vi "Cube Manipulation Logic Core.vi"(6 "Auto Control":bool, 8 "Manual Intake Control":dbl, 10 "Manual Lift Control":dbl, 11 "Cube Manipulation Button Controls":T3) -> (0 "Safety Limit Engaged":bool, 3 "output cluster":T1={"Control Mode"=1, "Carrage Output"=0.0, "Intake Output"=0.0, "Intake Short"=FALSE, "Intake Long"=FALSE, "Lift Output"=0.0} {"Control Mode" items=["PercentOutput"=0, "Position"=1, "Velocity"=2, "Current"=3, "Follower"=5, "MotionProfile"=6, "MotionMagic"=7, "MotionMagicArc"=8, "MotionProfileArc"=10, "Disabled"=15]}, 5 "Sequence Done":bool, 7 "Position Reached":bool)   [LabVIEW 2017]
uses:
  Cube Manipulation Controls.ctl
  Cube Manipulation Outputs.ctl
  <vilib>/Rock Robotics/WPI/ThirdParty/Phoenix-LabVIEW/Motor Controller/Controls/CTRE_Phoenix_MotorControl_ControlMode.ctl
  Robot Global Data.vi
panel:
  in  "Intake Output":dbl=0.75 format="%#_13g"
  in  "y":dbl=-3500.0 format="%#_13g"
  in  "Exchange Sequence":dbl
  in  "Trigger Offset":dbl=5000.0
  in  "Command":dbl
  in  "Sequence Position":dbl
  # "Off= Retracted\nOn= Extended"
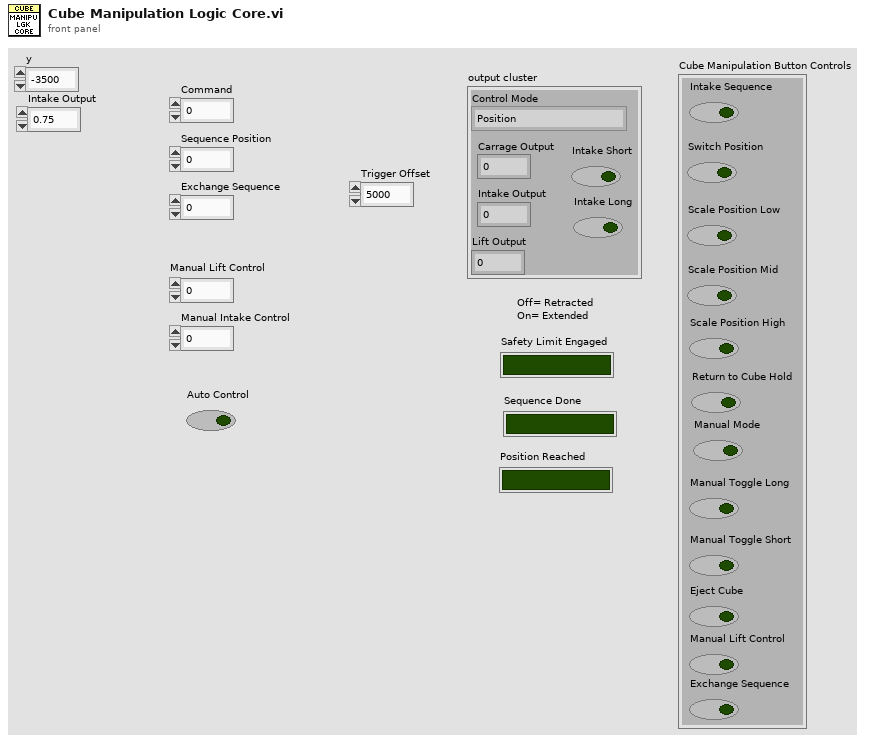
[diagram p1: front panel]
types:
  T1 = typedef "Cube Manipulation Outputs.ctl" = cluster{"Control Mode":T2, "Carrage Output":dbl, "Intake Output":dbl, "Intake Short":bool, "Intake Long":bool, "Lift Output":dbl}
  T2 = typedef "CTRE_Phoenix_MotorControl_ControlMode.ctl" = u16
  T3 = typedef "Cube Manipulation Controls.ctl" = cluster{"Intake Sequence":bool, "Switch Position":bool, "Scale Position Low":bool, "Scale Position Mid":bool, "Scale Position High":bool, "Return to Cube Hold":bool, "Manual Mode":bool, "Manual Toggle Long":bool, "Manual Toggle Short":bool, "Eject Cube":bool, "Manual Lift Control":bool, "Exchange Sequence":bool}
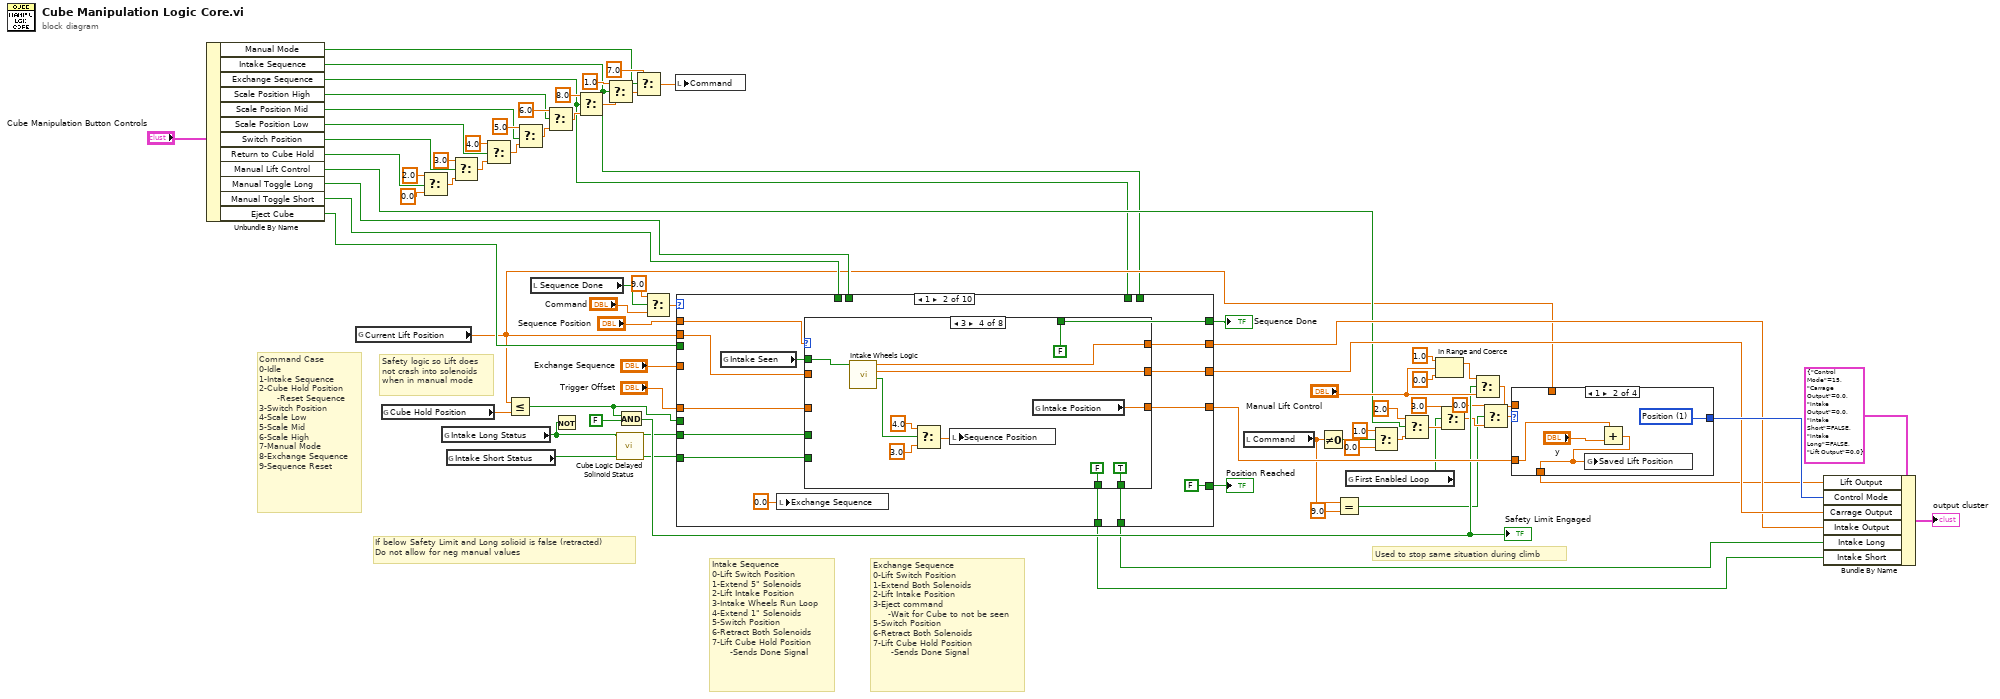
[diagram p0: block diagram]
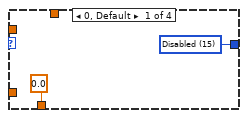
[diagram p2: hidden frame]
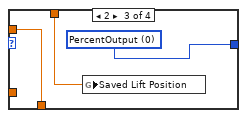
[diagram p3: hidden frame]
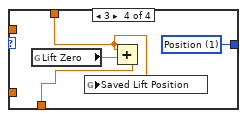
[diagram p4: hidden frame]
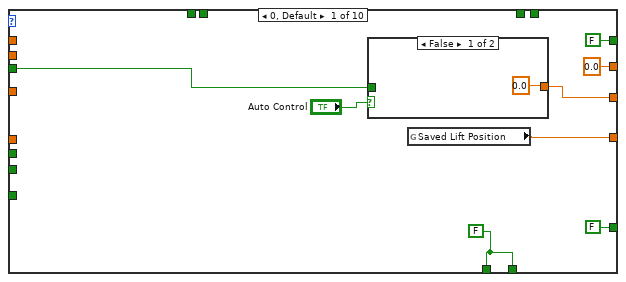
[diagram p5: hidden frame]
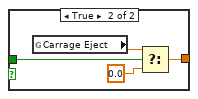
[diagram p6: hidden frame]
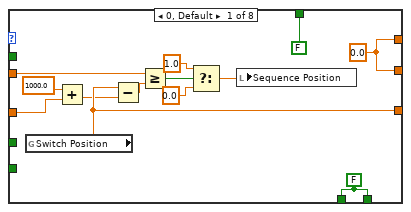
[diagram p7: hidden frame]
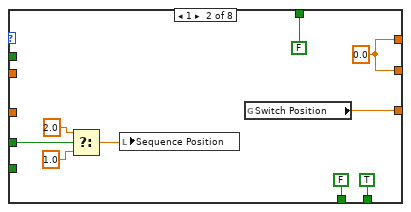
[diagram p8: hidden frame]
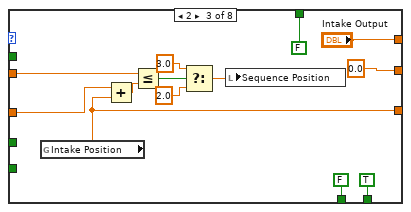
[diagram p9: hidden frame]
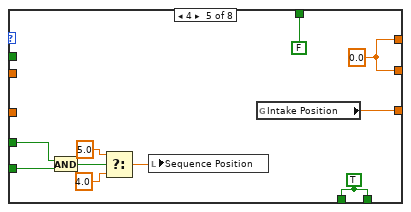
[diagram p10: hidden frame]
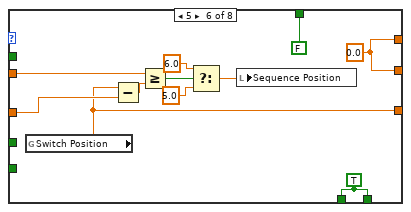
[diagram p11: hidden frame]
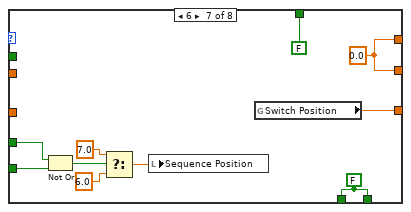
[diagram p12: hidden frame]
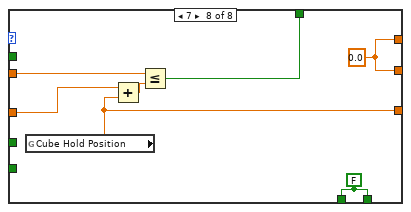
[diagram p13: hidden frame]
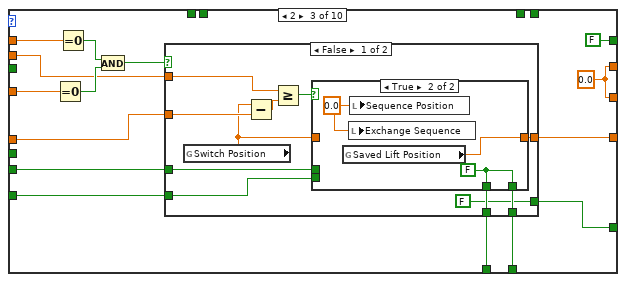
[diagram p14: hidden frame]
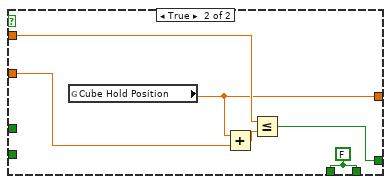
[diagram p16: hidden frame]
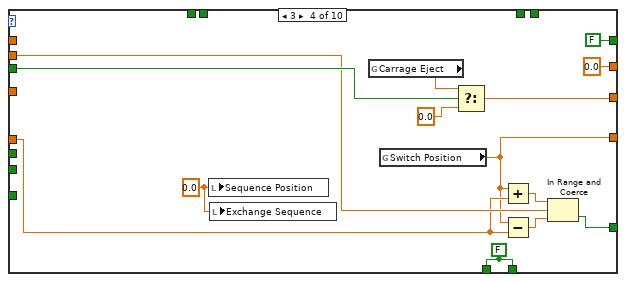
[diagram p17: hidden frame]
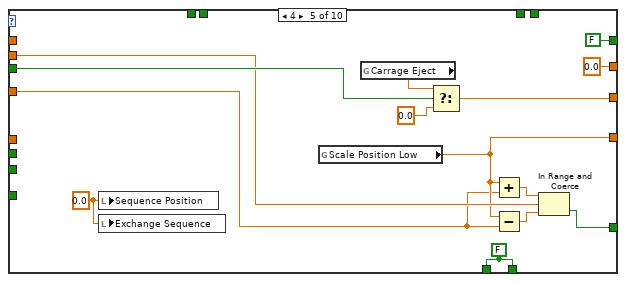
[diagram p18: hidden frame]
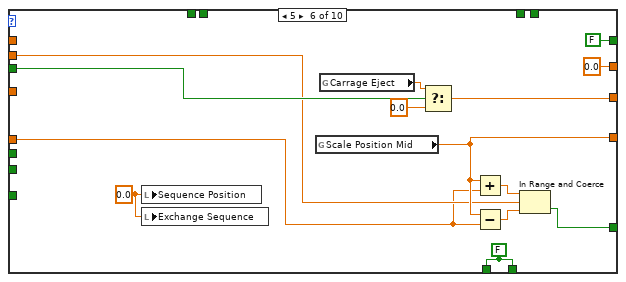
[diagram p19: hidden frame]
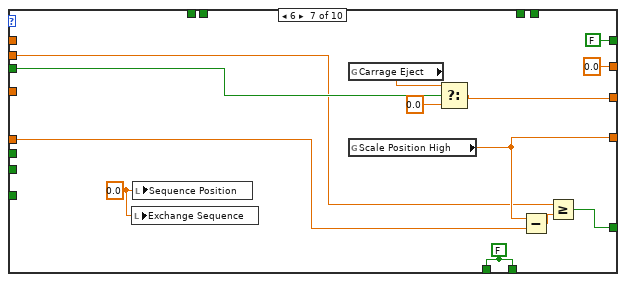
[diagram p20: hidden frame]
diagram:
  # "Used to stop same situation during climb"
  # "Exchange Sequence\n0-Lift Switch Position\n1-Extend Both Solenoids\n2-Lift Intake Position\n3-Eject command\n     -Wait for Cube to not be seen\n5-Switch Position\n6-Retract Both Solenoids\n7-Lift Cube Hold Position\n      -Sends Done Signal"
  # "If below Safety Limit and Long solioid is false (retracted)\nDo not allow for neg manual values"
  # "Command Case\n0-Idle\n1-Intake Sequence\n2-Cube Hold Position\n      -Reset Sequence\n3-Switch Position\n4-Scale Low\n5-Scale Mid\n6-Scale High\n7-Manual Mode\n8-Exchange Sequence\n9-Sequence Reset"
  # "Safety logic so Lift does\nnot crash into solenoids\nwhen in manual mode"
  # "Intake Sequence\n0-Lift Switch Position\n1-Extend 5\" Solenoids\n2-Lift Intake Position\n3-Intake Wheels Run Loop\n4-Extend 1\" Solenoids\n5-Switch Position\n6-Retract Both Solenoids\n7-Lift Cube Hold Position\n      -Sends Done Signal"
  n1 = Unbundle By Name("Cube Manipulation Button Controls") -> ("Manual Mode"=w29:bool, "Intake Sequence"=w21:bool, "Exchange Sequence"=w20:bool, "Scale Position High"=w45:bool, "Scale Position Mid"=w46:bool, "Scale Position Low"=w47:bool, "Switch Position"=w48:bool, "Return to Cube Hold"=w49:bool, "Manual Lift Control"=w34:bool, "Manual Toggle Long"=w36:bool, "Manual Toggle Short"=w35:bool, "Eject Cube"=w37:bool)
  n2 = global read "Robot Global Data.vi" "Current Lift Position"() -> (w33:dbl)
  n3 = global read "Robot Global Data.vi" "Cube Hold Position"() -> (w8:dbl)
  n4 = Select(t=2.0, s=w49, f=0.0) -> (s? t:f=w73:dbl)
  n5 = global read "Robot Global Data.vi" "Intake Long Status"() -> (w15:bool)
  n6 = global read "Robot Global Data.vi" "Intake Short Status"() -> (w14:bool)
  n7 = Select(t=3.0, s=w48, f=w73) -> (s? t:f=w74:dbl)
  n8 = Select(t=4.0, s=w47, f=w74) -> (s? t:f=w75:dbl)
  n9 = Less Or Equal?(x=w33, y=w8) -> (x <= y?=w9:bool)
  n10 = Select(t=5.0, s=w46, f=w75) -> (s? t:f=w72:dbl)
  n11 = local read "Sequence Done"() -> (w23:bool)
  n12 = Select(t=6.0, s=w45, f=w72) -> (s? t:f=w76:dbl)
  n13 = Not(x=w15) -> ()  [unwired: 1 out]
  n14 = Select(t=8.0, s=w20, f=w76) -> (s? t:f=w59:dbl)
  n15 = Select(t=1.0, s=w21, f=w59) -> (s? t:f=w32:dbl)
  n16 = call "Cube Logic Delayed Solinoid Status.vi"("Short Input"=w14, "Long Input"=w15) -> ("Short Delayed Output"=w16:bool, "Long Delayed Output"=w17:bool)  [unwired: 8 in]
  n17 = And(x=w9, y=FALSE) -> (x .and. y?=w44:bool)
  "Safety Limit Engaged" <- w44
  n18 = Select(t=7.0, s=w29, f=w32) -> (s? t:f=w31:dbl)
  n19 = Select(t=9.0, s=w23, f="Command") -> (s? t:f=w25:dbl)
  n20 = local write "Command"(w31) -> ()
  n21 = case shown="1" w25 {
    tunnel: w33 -> [_ w103 w190 w232 w244 w257 w270 _ w322 _]
    tunnel: [w81 w102 w196 w228 w243 w258 w272 w286 w321 w400] -> w57
    tunnel: [w77 w101 w195 w239 w253 w267 w280 w300 w320 w407] -> w19
    tunnel: [w77 w100 w194 w239 w253 w267 w280 w301 w319 w406] -> w18
    tunnel: w17 -> [_ w99 w192 _ _ _ _ _ w318 w407]
    tunnel: [0.0 ("Intake Output") w98 w188 0.0 ("Intake Output") 0.0 ("Intake Output") 0.0 ("Intake Output") 0.0 ("Intake Output") w297 w317 w399] -> w40
    tunnel: [w80 w97 w188 w237 w252 w266 w278 w299 w316 w399] -> w41
    tunnel: w16 -> [_ w95 w193 _ _ _ _ _ w315 w406]
    tunnel: "Sequence Position" -> [_ w94 w200 _ _ _ _ _ _ _]
    tunnel: w37 -> [w79 _ _ w238 w251 w264 w277 _ w309 _]
    tunnel: w36 -> [_ _ _ _ _ _ _ w282 _ _]
    tunnel: w35 -> [_ _ _ _ _ _ _ w281 _ _]
    tunnel: "Trigger Offset" -> [_ w93 w191 w229 _ w256 w271 _ w314 _]
    tunnel: "Exchange Sequence" -> [_ _ w201 _ w242 _ _ _ w313 _]
    tunnel: [FALSE w92 FALSE FALSE FALSE FALSE FALSE FALSE w312 w404] -> w26
    tunnel: w21 -> [_ _ _ _ _ _ _ _ _ w403]
    tunnel: w20 -> [_ _ _ _ _ _ _ _ _ w402]
    tunnel: [FALSE FALSE w189 w233 w245 w259 w273 FALSE FALSE FALSE] -> w13
    tunnel: w9 -> [_ _ _ _ _ _ _ _ _ _]
    frame 0, Default {
      w77 = FALSE
      n22 = case shown="False" "Auto Control" {
        tunnel: [0.0 w87] -> w80
        tunnel: w79 -> [_ w86]
        frame False {
        }
        frame True {
          n23 = global read "Robot Global Data.vi" "Carrage Eject"() -> (w89:dbl)
          n24 = Select(t=w89, s=w86, f=0.0) -> (s? t:f=w87:dbl)
        }
      }
      n25 = global read "Robot Global Data.vi" "Saved Lift Position"() -> (w81:dbl)
    }
    frame 1 {
      n26 = global read "Robot Global Data.vi" "Intake Seen"() -> (w96:bool)
      n27 = local write "Exchange Sequence"(0.0 ("Exchange Sequence")) -> ()
      n28 = case shown="3" w94 {
        tunnel: w103 -> [w116 _ w133 _ _ w170 _ w187]
        tunnel: [w109 w125 w130 w147 w159 w163 w180 w184] -> w102
        tunnel: w93 -> [w110 _ w129 _ _ w164 _ w183]
        tunnel: [w108 TRUE TRUE TRUE w158 w162 w179 w185] -> w101
        tunnel: [w108 FALSE FALSE FALSE w158 w162 w179 w185] -> w100
        tunnel: w99 -> [_ w120 _ _ w153 _ w173 _]
        tunnel: [w106 w117 "Intake Output" w142 w150 w160 w171 w181] -> w98
        tunnel: [w106 w117 0.0 ("Intake Output") w141 w150 w160 w171 w181] -> w97
        tunnel: w96 -> [_ _ _ w140 _ _ _ _]
        tunnel: w95 -> [_ _ _ _ w152 _ w175 _]
        tunnel: [FALSE FALSE FALSE FALSE FALSE FALSE FALSE w182] -> w92
        frame 0, Default {
          w106 = 0.0 ("Intake Output")
          w108 = FALSE
          n29 = global read "Robot Global Data.vi" "Switch Position"() -> (w109:dbl)
          n30 = Add(x=1000.0, y=w110) -> (x+y=w105:dbl)
          n31 = Subtract(x=w109, y=w105) -> (x-y=w111:dbl)
          n32 = Greater Or Equal?(x=w116, y=w111) -> (x >= y?=w115:bool)
          n33 = Select(t=1.0, s=w115, f=0.0) -> (s? t:f=w112:dbl)
          n34 = local write "Sequence Position"(w112) -> ()
        }
        frame 1 {
          w117 = 0.0 ("Intake Output")
          n35 = Select(t=2.0, s=w120, f=1.0) -> (s? t:f=w119:dbl)
          n36 = local write "Sequence Position"(w119) -> ()
          n37 = global read "Robot Global Data.vi" "Switch Position"() -> (w125:dbl)
        }
        frame 2 {
          n38 = global read "Robot Global Data.vi" "Intake Position"() -> (w130:dbl)
          n39 = Add(x=w129, y=w130) -> (x+y=w134:dbl)
          n40 = Less Or Equal?(x=w133, y=w134) -> (x <= y?=w136:bool)
          n41 = Select(t=3.0, s=w136, f=2.0) -> (s? t:f=w131:dbl)
          n42 = local write "Sequence Position"(w131) -> ()
        }
        frame 3 {
          n43 = call "Intake Wheels Logic.vi"("Intake Seen"=w140) -> ("Done"=w144:bool, "Carrage Output"=w141:dbl, "Intake Output"=w142:dbl)  [unwired: 8 in]
          n44 = Select(t=4.0, s=w144, f=3.0) -> (s? t:f=w143:dbl)
          n45 = local write "Sequence Position"(w143) -> ()
          n46 = global read "Robot Global Data.vi" "Intake Position"() -> (w147:dbl)
        }
        frame 4 {
          w158 = TRUE
          w150 = 0.0 ("Intake Output")
          n47 = And(x=w153, y=w152) -> (x .and. y?=w154:bool)
          n48 = Select(t=5.0, s=w154, f=4.0) -> (s? t:f=w155:dbl)
          n49 = local write "Sequence Position"(w155) -> ()
          n50 = global read "Robot Global Data.vi" "Intake Position"() -> (w159:dbl)
        }
        frame 5 {
          w160 = 0.0 ("Intake Output")
          w162 = TRUE
          n51 = global read "Robot Global Data.vi" "Switch Position"() -> (w163:dbl)
          n52 = Subtract(x=w163, y=w164) -> (x-y=w165:dbl)
          n53 = Greater Or Equal?(x=w170, y=w165) -> (x >= y?=w169:bool)
          n54 = Select(t=6.0, s=w169, f=5.0) -> (s? t:f=w166:dbl)
          n55 = local write "Sequence Position"(w166) -> ()
        }
        frame 6 {
          w179 = FALSE
          w171 = 0.0 ("Intake Output")
          n56 = Not Or(1:w175, 2:w173) -> (0:w174:bool)
          n57 = Select(t=7.0, s=w174, f=6.0) -> (s? t:f=w176:dbl)
          n58 = local write "Sequence Position"(w176) -> ()
          n59 = global read "Robot Global Data.vi" "Switch Position"() -> (w180:dbl)
        }
        frame 7 {
          w181 = 0.0 ("Intake Output")
          w185 = FALSE
          n60 = global read "Robot Global Data.vi" "Cube Hold Position"() -> (w184:dbl)
          n61 = Add(x=w183, y=w184) -> (x+y=w186:dbl)
          n62 = Less Or Equal?(x=w187, y=w186) -> (x <= y?=w182:bool)
        }
      }
    }
    frame 2 {
      w188 = 0.0 ("Intake Output")
      n63 = Equal To 0?(x=w201) -> (x = 0?=w198:bool)
      n64 = Equal To 0?(x=w200) -> (x = 0?=w199:bool)
      n65 = And(x=w199, y=w198) -> (x .and. y?=w197:bool)
      n66 = case shown="False" w197 {
        tunnel: [w206 w222] -> w196
        tunnel: [w208 w225] -> w195
        tunnel: [w209 w225] -> w194
        tunnel: w193 -> [w205 _]
        tunnel: w192 -> [w204 _]
        tunnel: w191 -> [w212 w221]
        tunnel: w190 -> [w211 w223]
        tunnel: [FALSE w220] -> w189
        frame False {
          n67 = global read "Robot Global Data.vi" "Switch Position"() -> (w207:dbl)
          n68 = Subtract(x=w207, y=w212) -> (x-y=w213:dbl)
          n69 = Greater Or Equal?(x=w211, y=w213) -> (x >= y?=w210:bool)
          n70 = case shown="True" w210 {
            tunnel: [w215 w219] -> w209
            tunnel: [w214 w219] -> w208
            tunnel: w207 -> [w216 _]
            tunnel: [w216 w217] -> w206
            tunnel: w205 -> [w215 _]
            tunnel: w204 -> [w214 _]
            frame False {
            }
            frame True {
              w218 = 0.0 ("Sequence Position")
              w219 = FALSE
              n71 = global read "Robot Global Data.vi" "Saved Lift Position"() -> (w217:dbl)
              n72 = local write "Exchange Sequence"(w218) -> ()
              n73 = local write "Sequence Position"(w218) -> ()
            }
          }
        }
        frame True {
          w225 = FALSE
          n74 = global read "Robot Global Data.vi" "Cube Hold Position"() -> (w222:dbl)
          n75 = Add(x=w222, y=w221) -> (x+y=w224:dbl)
          n76 = Less Or Equal?(x=w223, y=w224) -> (x <= y?=w220:bool)
        }
      }
    }
    frame 3 {
      w234 = 0.0 ("Sequence Position")
      w239 = FALSE
      n77 = local write "Sequence Position"(w234) -> ()
      n78 = local write "Exchange Sequence"(w234) -> ()
      n79 = global read "Robot Global Data.vi" "Carrage Eject"() -> (w226:dbl)
      n80 = global read "Robot Global Data.vi" "Switch Position"() -> (w228:dbl)
      n81 = Select(t=w226, s=w238, f=0.0 ("t")) -> (s? t:f=w237:dbl)
      n82 = Add(x=w228, y=w229) -> (x+y=w231:dbl)
      n83 = Subtract(x=w228, y=w229) -> (x-y=w230:dbl)
      n84 = In Range and Coerce(upper limit=w231, x=w232, lower limit=w230) -> (In Range?=w233:bool)  [unwired: 1 out]
    }
    frame 4 {
      w248 = 0.0 ("Sequence Position")
      w253 = FALSE
      n85 = local write "Sequence Position"(w248) -> ()
      n86 = local write "Exchange Sequence"(w248) -> ()
      n87 = global read "Robot Global Data.vi" "Scale Position Low"() -> (w243:dbl)
      n88 = global read "Robot Global Data.vi" "Carrage Eject"() -> (w240:dbl)
      n89 = Select(t=w240, s=w251, f=0.0 ("t")) -> (s? t:f=w252:dbl)
      n90 = Add(x=w243, y=w242) -> (x+y=w247:dbl)
      n91 = Subtract(x=w243, y=w242) -> (x-y=w246:dbl)
      n92 = In Range and Coerce(upper limit=w247, x=w244, lower limit=w246) -> (In Range?=w245:bool)  [unwired: 1 out]
    }
    frame 5 {
      w262 = 0.0 ("Sequence Position")
      w267 = FALSE
      n93 = local write "Sequence Position"(w262) -> ()
      n94 = local write "Exchange Sequence"(w262) -> ()
      n95 = global read "Robot Global Data.vi" "Scale Position Mid"() -> (w258:dbl)
      n96 = global read "Robot Global Data.vi" "Carrage Eject"() -> (w255:dbl)
      n97 = Select(t=w255, s=w264, f=0.0) -> (s? t:f=w266:dbl)
      n98 = Add(x=w258, y=w256) -> (x+y=w261:dbl)
      n99 = Subtract(x=w258, y=w256) -> (x-y=w260:dbl)
      n100 = In Range and Coerce(upper limit=w261, x=w257, lower limit=w260) -> (In Range?=w259:bool)  [unwired: 1 out]
    }
    frame 6 {
      w275 = 0.0 ("Sequence Position")
      w280 = FALSE
      n101 = local write "Exchange Sequence"(w275) -> ()
      n102 = local write "Sequence Position"(w275) -> ()
      n103 = global read "Robot Global Data.vi" "Carrage Eject"() -> (w269:dbl)
      n104 = global read "Robot Global Data.vi" "Scale Position High"() -> (w272:dbl)
      n105 = Select(t=w269, s=w277, f=0.0) -> (s? t:f=w278:dbl)
      n106 = Subtract(x=w272, y=w271) -> (x-y=w274:dbl)
      n107 = Greater Or Equal?(x=w270, y=w274) -> (x >= y?=w273:bool)
    }
    frame 7 {
      w288 = 0.0 ("Sequence Position")
      # "Long"
      # "Short"
      n108 = local write "Sequence Position"(w288) -> ()
      n109 = local write "Exchange Sequence"(w288) -> ()
      n110 = case shown="False" w281 {
        tunnel: [w305 w306] -> w301
        frame False {
          n111 = global read "Robot Global Data.vi" "Intake Short Status"() -> (w305:bool)
        }
        frame True {
          n112 = global read "Robot Global Data.vi" "Intake Short Status"() -> (w307:bool)
          n113 = Not(x=w307) -> (.not. x?=w306:bool)
          n114 = global write "Robot Global Data.vi" "Intake Short Status"(w306) -> ()
        }
      }
      n115 = case shown="True" w282 {
        tunnel: [w302 w303] -> w300
        frame False {
          n116 = global read "Robot Global Data.vi" "Intake Long Status"() -> (w302:bool)
        }
        frame True {
          n117 = global read "Robot Global Data.vi" "Intake Long Status"() -> (w304:bool)
          n118 = Not(x=w304) -> (.not. x?=w303:bool)
          n119 = global write "Robot Global Data.vi" "Intake Long Status"(w303) -> ()
        }
      }
      n120 = Less?(x="Manual Intake Control", y=-0.25) -> (x < y?=w293:bool)
      n121 = Greater?(x="Manual Intake Control", y=0.25) -> (0:w294:bool)
      n122 = global read "Robot Global Data.vi" "Saved Lift Position"() -> (w286:dbl)
      n123 = global read "Robot Global Data.vi" "Carrage Intake"() -> (w284:dbl)
      n124 = global read "Robot Global Data.vi" "Carrage Eject"() -> (w283:dbl)
      n125 = Select(t=1.0, s=w294, f=0.0) -> (s? t:f=w297:dbl)
      n126 = Select(t=w284, s=w294, f=0.0) -> (s? t:f=w298:dbl)
      n127 = Select(t=w283, s=w293, f=w298) -> (s? t:f=w299:dbl)
    }
    frame 8 {
      n128 = global read "Robot Global Data.vi" "Intake Seen"() -> (w310:bool)
      n129 = local write "Sequence Position"(0.0 ("Sequence Position")) -> ()
      n130 = case shown="5" w313 {
        tunnel: w322 -> [w333 _ w351 _ w381 _ w398]
        tunnel: [w326 w343 w348 w367 w375 w391 w395] -> w321
        tunnel: w314 -> [w327 _ w347 _ w371 _ w394]
        tunnel: [w325 w342 w346 TRUE w374 w390 w396] -> w320
        tunnel: [w325 w342 w346 FALSE w374 w390 w396] -> w319
        tunnel: w318 -> [_ w336 _ _ _ w384 _]
        tunnel: [w323 w334 w344 w362 w372 w382 w392] -> w317
        tunnel: [w323 w334 w344 w363 w372 w382 w392] -> w316
        tunnel: w315 -> [_ w338 _ _ _ w386 _]
        tunnel: [FALSE FALSE FALSE FALSE FALSE FALSE w393] -> w312
        tunnel: w310 -> [_ _ _ w364 _ _ _]
        tunnel: w309 -> [_ _ _ w359 _ _ _]
        frame 0, Default {
          w323 = 0.0 ("Intake Output")
          w325 = FALSE
          n131 = global read "Robot Global Data.vi" "Switch Position"() -> (w326:dbl)
          n132 = Subtract(x=w326, y=w327) -> (x-y=w328:dbl)
          n133 = Greater Or Equal?(x=w333, y=w328) -> (x >= y?=w332:bool)
          n134 = Select(t=1.0, s=w332, f=0.0) -> (s? t:f=w329:dbl)
          n135 = local write "Exchange Sequence"(w329) -> ()
        }
        frame 1 {
          w342 = TRUE
          w334 = 0.0 ("Intake Output")
          n136 = And(x=w336, y=w338) -> (x .and. y?=w337:bool)
          n137 = Select(t=2.0, s=w337, f=1.0) -> (s? t:f=w339:dbl)
          n138 = local write "Exchange Sequence"(w339) -> ()
          n139 = global read "Robot Global Data.vi" "Switch Position"() -> (w343:dbl)
        }
        frame 2 {
          w344 = 0.0 ("Intake Output")
          w346 = TRUE
          n140 = global read "Robot Global Data.vi" "Intake Position"() -> (w348:dbl)
          n141 = Add(x=w347, y=w348) -> (x+y=w352:dbl)
          n142 = Less Or Equal?(x=w351, y=w352) -> (x <= y?=w354:bool)
          n143 = Select(t=3.0, s=w354, f=2.0) -> (s? t:f=w349:dbl)
          n144 = local write "Exchange Sequence"(w349) -> ()
        }
        frame 3 {
          n145 = Not(x=w364) -> (.not. x?=w358:bool)
          n146 = Select(t=5.0, s=w358, f=3.0) -> (s? t:f=w368:dbl)
          n147 = global read "Robot Global Data.vi" "Carrage Eject"() -> (w357:dbl)
          n148 = local write "Exchange Sequence"(w368) -> ()
          n149 = global read "Robot Global Data.vi" "Intake Position"() -> (w367:dbl)
          n150 = Select(t=w357, s=w359, f=0.0) -> (s? t:f=w363:dbl)
          n151 = Select(t=-1.0 ("Intake Output"), s=w359, f=0.0) -> (s? t:f=w362:dbl)
        }
        frame 5 {
          w372 = 0.0 ("Intake Output")
          w374 = TRUE
          n152 = global read "Robot Global Data.vi" "Switch Position"() -> (w375:dbl)
          n153 = Subtract(x=w375, y=w371) -> (x-y=w376:dbl)
          n154 = Greater Or Equal?(x=w381, y=w376) -> (x >= y?=w380:bool)
          n155 = Select(t=6.0, s=w380, f=5.0) -> (s? t:f=w377:dbl)
          n156 = local write "Exchange Sequence"(w377) -> ()
        }
        frame 6 {
          w390 = FALSE
          w382 = 0.0 ("Intake Output")
          n157 = Not Or(1:w386, 2:w384) -> (0:w385:bool)
          n158 = Select(t=7.0, s=w385, f=6.0) -> (s? t:f=w387:dbl)
          n159 = local write "Exchange Sequence"(w387) -> ()
          n160 = global read "Robot Global Data.vi" "Switch Position"() -> (w391:dbl)
        }
        frame 7 {
          w392 = 0.0 ("Intake Output")
          w396 = FALSE
          n161 = global read "Robot Global Data.vi" "Cube Hold Position"() -> (w395:dbl)
          n162 = Add(x=w394, y=w395) -> (x+y=w397:dbl)
          n163 = Less Or Equal?(x=w398, y=w397) -> (x <= y?=w393:bool)
        }
      }
    }
    frame 9 {
      w405 = 0.0 ("Sequence Position")
      w399 = 0.0 ("Intake Output")
      n164 = local write "Sequence Position"(w405) -> ()
      n165 = local write "Exchange Sequence"(w405) -> ()
      n166 = global read "Robot Global Data.vi" "Cube Hold Position"() -> (w400:dbl)
      n167 = Or(x=w403, y=w402) -> (x .or. y?=w404:bool)
    }
  }
  "Sequence Done" <- w26
  "Position Reached" <- w13
  n168 = local read "Command"() -> (w5:dbl)
  n169 = Not Equal To 0?(x=w5) -> (x != 0?=w62:bool)
  n170 = Equal?(x=w5, y=9.0) -> (x = y?=w3:bool)
  n171 = global read "Robot Global Data.vi" "First Enabled Loop"() -> (w10:bool)
  n172 = Select(t=1.0, s=w62, f=0.0) -> (s? t:f=w64:dbl)
  n173 = Select(t=2.0, s=w34, f=w64) -> (s? t:f=w12:dbl)
  n174 = In Range and Coerce(upper limit=1.0, x="Manual Lift Control", lower limit=0.0) -> (coerced(x)=w53:dbl)  [unwired: 1 out]
  n175 = Select(t=3.0, s=w10, f=w12) -> (s? t:f=w6:dbl)
  n176 = Select(t=w53, s=w44, f="Manual Lift Control") -> (s? t:f=w54:dbl)
  n177 = Select(t=0.0, s=w3, f=w6) -> (s? t:f=w7:dbl)
  n178 = case shown="1" w7 {
    tunnel: w54 -> [_ _ w415 _]
    tunnel: w57 -> [_ w411 _ _]
    tunnel: w33 -> [_ _ w414 w417]
    tunnel: [w409 w413 w416 w420] -> w42
    tunnel: [0.0 ("Current Lift Position") w412 w415 w418] -> w38
    frame 0, Default {
      w409 = T2 15 items=["PercentOutput"=0, "Position"=1, "Velocity"=2, "Current"=3, "Follower"=5, "MotionProfile"=6, "MotionMagic"=7, "MotionMagicArc"=8, "MotionProfileArc"=10, "Disabled"=15] ("Control Mode")
    }
    frame 1 {
      w413 = T2 1 items=["PercentOutput"=0, "Position"=1, "Velocity"=2, "Current"=3, "Follower"=5, "MotionProfile"=6, "MotionMagic"=7, "MotionMagicArc"=8, "MotionProfileArc"=10, "Disabled"=15] ("Control Mode")
      n179 = Add(x=w411, y="y") -> (x+y=w412:dbl)
      n180 = global write "Robot Global Data.vi" "Saved Lift Position"(w412) -> ()
    }
    frame 2 {
      w416 = T2 0 items=["PercentOutput"=0, "Position"=1, "Velocity"=2, "Current"=3, "Follower"=5, "MotionProfile"=6, "MotionMagic"=7, "MotionMagicArc"=8, "MotionProfileArc"=10, "Disabled"=15] ("Control Mode")
      n181 = global write "Robot Global Data.vi" "Saved Lift Position"(w414) -> ()
    }
    frame 3 {
      w420 = T2 1 items=["PercentOutput"=0, "Position"=1, "Velocity"=2, "Current"=3, "Follower"=5, "MotionProfile"=6, "MotionMagic"=7, "MotionMagicArc"=8, "MotionProfileArc"=10, "Disabled"=15] ("Control Mode")
      n182 = global read "Robot Global Data.vi" "Lift Zero"() -> (w419:dbl)
      n183 = global write "Robot Global Data.vi" "Saved Lift Position"(w417) -> ()
      n184 = Add(x=w417, y=w419) -> (x+y=w418:dbl)
    }
  }
  n185 = Bundle By Name(cluster=T1 {"Control Mode"=15, "Carrage Output"=0.0, "Intake Output"=0.0, "Intake Short"=FALSE, "Intake Long"=FALSE, "Lift Output"=0.0}, "Lift Output"=w38, "Control Mode"=w42, "Carrage Output"=w41, "Intake Output"=w40, "Intake Long"=w19, "Intake Short"=w18) -> (→"output cluster":T1)
